vi "uart.vi"() -> ()   [LabVIEW 2018]
uses:
  <vilib>/Instr/_visa.llb/VISA Configure Serial Port (Instr).vi
panel:
  in  "speed 4":string
  in  "speed 3":string
  in  "speed 2":string
  in  "speed 1":string
  in  "Length of individual speed command (including sign)":i32=8
  in  "Number of Motors to control":i32=4
  out "Array":dbl[](array[numeric])=[-8.7767705, 5.7767688, 88.776768, 80.776768]
  out "concatenated string":string="8.7767685.7767688.7767680.776768-8.7767705.7767688.7767680.776768-8.7767705.7767688.7767680.776768-8.7767705.7767688.7767680.776768-8.7767705.7767688.7767680.776768-8.7767705.7767688.7767680.776768"
  in  "timeout (10sec)":u32=10000
  in  "stop":bool
  # "Write the indivual speeds here, noting that you must include the\n+ sign for positive values, and - for negative values:\n\ne.g.\n+0.232\n-0.234\n+0.254\n-0.233"
  # "output"
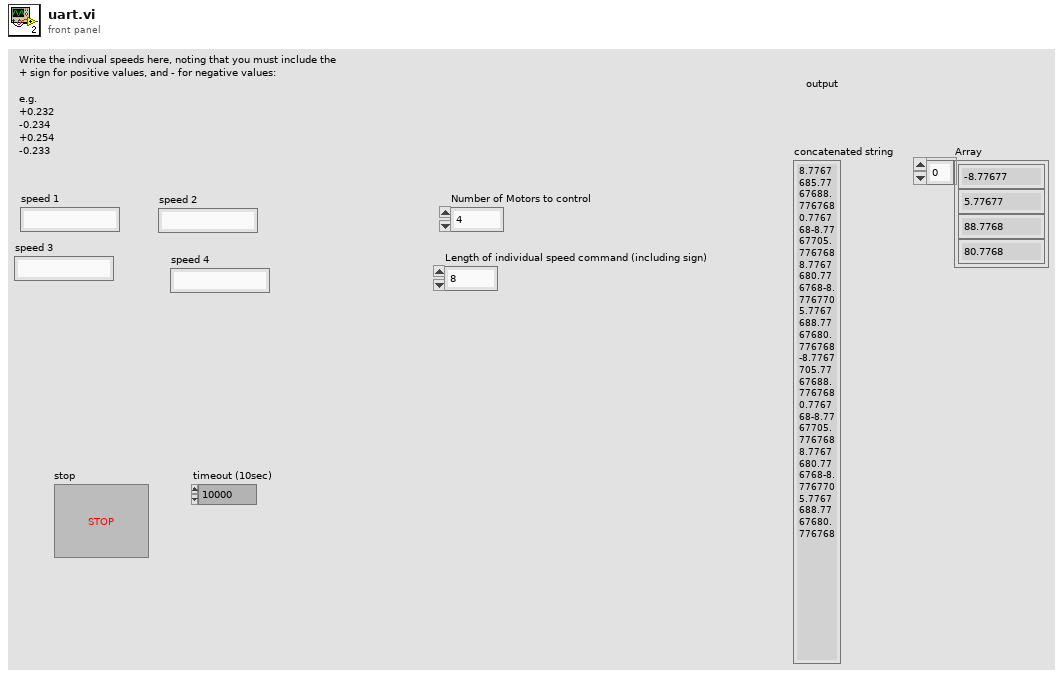
[diagram p1: front panel]
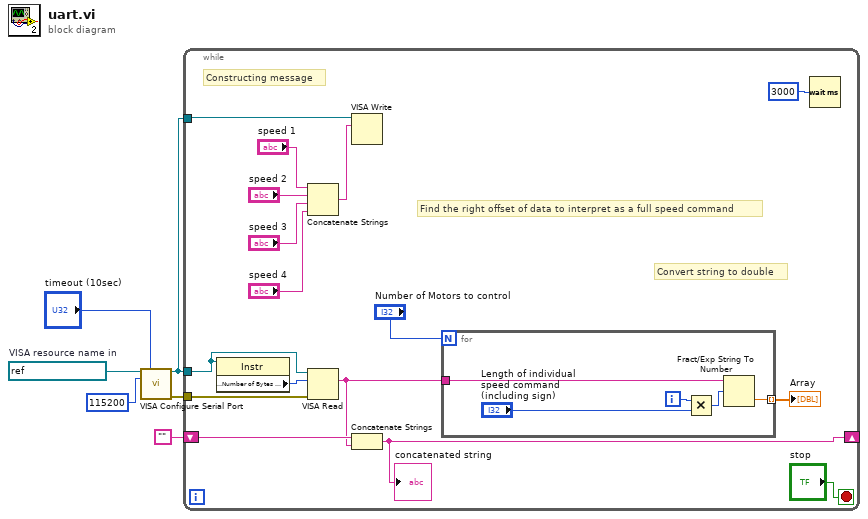
[diagram p0: block diagram]
diagram:
  w6 = refnum<visa-resource-name> "ASRL2::INSTR"  # VISA resource name in
  n1 = call-poly "VISA Configure Serial Port"("VISA resource name"=w6, "timeout (10sec)"="timeout (10sec)", "baud rate (9600)"=u32 115200) -> ("VISA resource name out"=w2:refnum<visa-resource-name>, "error out"=w1:errorcluster)  [unwired: 11 in]
  n2 = while {
    tunnel: w2 -> [w21]
    shift-right: [w15] -> _
    shift-left: "" -> [w19]
    tunnel: w2 -> [w18]
    tunnel: w1 -> [w17]
    stop <- "stop" stop-if-true
    # "Convert string to double"
    # "Find the right offset of data to interpret as a full speed command"
    # "Constructing message"
    n3 = property class="Instr"(reference=w21) -> ("Serial Settings:Number of Bytes at Serial Port"=w20:u32)  [unwired: 1 in, 2 out]
    n4 = Concatenate Strings("speed 1", "speed 2", "speed 3", "speed 4") -> (w14:string)
    n5 = VISA Read(VISA resource name=w21, byte count=w20, error in (no error)=w17) -> (read buffer=w12:string)  [unwired: 3 out]
    n6 = VISA Write(VISA resource name=w18, write buffer=w14) -> ()  [unwired: 1 in, 3 out]
    n7 = Concatenate Strings(w19, w12) -> (w15:string)
    "concatenated string" <- w15
    n8 = for {
      N: "Number of Motors to control" -> [_]
      tunnel: [w27] -> w13 mode=indexing
      tunnel: w12 -> [w24]
      i -> [w23]
      n9 = Multiply(x=w23, y="Length of individual speed command (including sign)") -> (x*y=w26:i32)
      n10 = Fract/Exp String To Number(string=w24, offset=w26) -> (number=w27:dbl)  [unwired: 2 in, 1 out]
    }
    "Array" <- w13
    n11 = Wait (ms)(milliseconds to wait=u32 3000) -> ()  [unwired: 1 out]
  }
